vi "StreamReceiveAcquisitionChD.vi"() -> ()   [LabVIEW 2018]
uses:
  <resource>/objmgr/ni.dex.rc
panel:
  in  "stop 2":bool
  out "error out 3":errorcluster
  out "error out":errorcluster
  in  "stop":bool
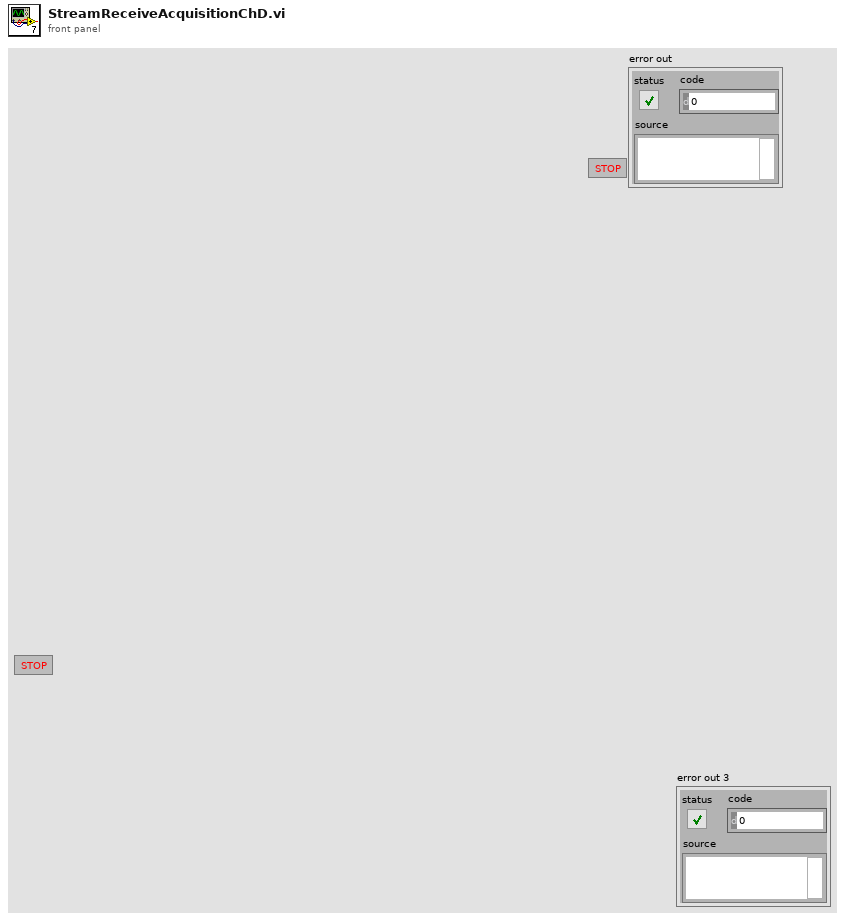
[diagram p1: front panel]
types:
  T1 = enum16{"Standard", "Buffered", "CRLF", "Immediate"}
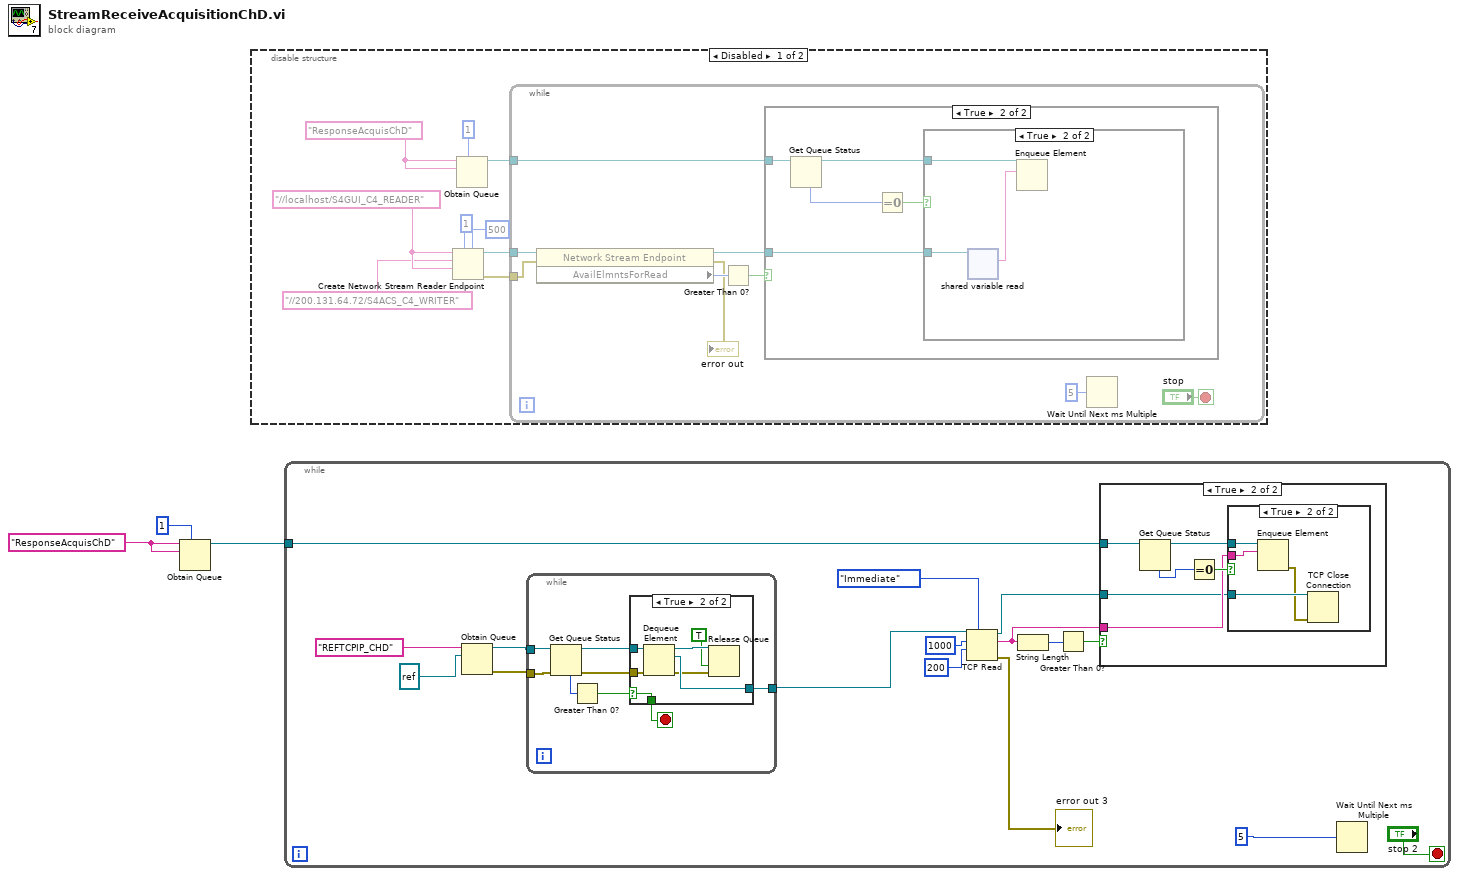
[diagram p0: block diagram]
diagram:
  w1 = "ResponseAcquisChD"
  n1 = Obtain Queue(max queue size (-1, unlimited)=1, name (unnamed)=w1, element data type=w1) -> (queue out=w3:refnum<queue>)  [unwired: 2 in, 2 out]
  n2 = disable-structure shown="Disabled" {
    frame Disabled {
      w7 = "//localhost/S4GUI_C4_READER"
      w12 = "ResponseAcquisChD"
      n3 = Create Network Stream Reader Endpoint(5:500 ("timeout in ms (-1)"), 7:1 ("reader buffer size"), 9:w7, 10:"//200.131.64.72/S4ACS_C4_WRITER", 11:w7) -> (0:w4:errorcluster, 3:w9:refnum<k21>)  [unwired: 2 in]
      n4 = Obtain Queue(max queue size (-1, unlimited)=1, name (unnamed)=w12, element data type=w12) -> (queue out=w11:refnum<queue>)  [unwired: 2 in, 2 out]
      n5 = while {
        tunnel: w11 -> [w20]
        tunnel: w9 -> [w19]
        tunnel: w4 -> [w14]
        stop <- "stop" stop-if-true
        n6 = property class="Network Stream Endpoint"(reference=w19, error in=w14) -> (reference out=w18:refnum<k21>, error out=→"error out":errorcluster, "AvailElmntsForRead"=w17:i32)
        n7 = Greater Than 0?(x=w17) -> (x > 0?=w16:bool)
        n8 = case shown="True" w16 {
          tunnel: w20 -> [_ w23]
          tunnel: w18 -> [_ w26]
          frame False {
          }
          frame True {
            n9 = Get Queue Status(queue=w23) -> (queue out=w22:refnum<queue>, # elements in queue=w25:i32)  [unwired: 2 in, 6 out]
            n10 = Equal To 0?(x=w25) -> (x = 0?=w24:bool)
            n11 = case shown="True" w24 {
              tunnel: w26 -> [_ w29]
              tunnel: w22 -> [_ w27]
              frame False {
              }
              frame True {
                n12 = shared-variable-read(w29) -> (w28:string)  [unwired: 2 in, 3 out]
                n13 = Enqueue Element(queue=w27, element=w28) -> ()  [unwired: 2 in, 3 out]
              }
            }
          }
        }
        n14 = Wait Until Next ms Multiple(millisecond multiple=u32 5) -> ()  [unwired: 1 out]
      }
    }
    frame Enabled {
    }
  }
  n15 = while {
    tunnel: w3 -> [w44]
    stop <- "stop 2" stop-if-true
    n16 = Obtain Queue(name (unnamed)="REFTCPIP_CHD", element data type=refnum<k5> refnum ("connection ID out")) -> (queue out=w31:refnum<queue>, error out=w30:errorcluster)  [unwired: 3 in, 1 out]
    n17 = while {
      tunnel: [w48] -> w34
      tunnel: w31 -> [w47]
      tunnel: w30 -> [w46]
      stop <- w49 stop-if-true
      n18 = Get Queue Status(queue=w47, error in (no error)=w46) -> (queue out=w53:refnum<queue>, error out=w52:errorcluster, # elements in queue=w50:i32)  [unwired: 1 in, 5 out]
      n19 = Greater Than 0?(x=w50) -> (x > 0?=w51:bool)
      n20 = case shown="True" w51 {
        selector: w51 -> [w54 w59]
        tunnel: w53 -> [_ w61]
        tunnel: w52 -> [_ w60]
        tunnel: [w54 w59] -> w49
        tunnel: [_ w58] -> w48
        frame False {
        }
        frame True {
          n21 = Dequeue Element(queue=w61, error in (no error)=w60) -> (queue out=w57:refnum<queue>, element=w58:refnum<k5>, error out=w56:errorcluster)  [unwired: 1 in, 1 out]
          n22 = Release Queue(queue=w57, force destroy? (F)=TRUE, error in (no error)=w56) -> ()  [unwired: 3 out]
        }
      }
    }
    n23 = TCP Read(connection ID=w34, bytes to read=1000, 7:T1."Immediate" ("mode (standard)"), 9:200 ("bytes to read")) -> (connection ID out=w35:refnum<k5>, data out=w40:string, error out=→"error out 3":errorcluster)  [unwired: 1 in]
    n24 = String Length(string=w40) -> (length=w42:i32)
    n25 = Greater Than 0?(x=w42) -> (x > 0?=w41:bool)
    n26 = case shown="True" w41 {
      tunnel: w44 -> [_ w65]
      tunnel: w40 -> [_ w63]
      tunnel: w35 -> [_ w62]
      frame False {
      }
      frame True {
        n27 = Get Queue Status(queue=w65) -> (queue out=w64:refnum<queue>, # elements in queue=w67:i32)  [unwired: 2 in, 6 out]
        n28 = Equal To 0?(x=w67) -> (x = 0?=w66:bool)
        n29 = case shown="True" w66 {
          tunnel: w64 -> [_ w71]
          tunnel: w63 -> [_ w70]
          tunnel: w62 -> [_ w69]
          frame False {
          }
          frame True {
            n30 = Enqueue Element(queue=w71, element=w70) -> (error out=w68:errorcluster)  [unwired: 2 in, 2 out]
            n31 = TCP Close Connection(connection ID=w69, error in (no error)=w68) -> ()  [unwired: 1 in, 2 out]
          }
        }
      }
    }
    n32 = Wait Until Next ms Multiple(millisecond multiple=u32 5) -> ()  [unwired: 1 out]
  }
